vi "ULx Write (Analog 1D DBL 1Chan 1Samp).vi"(0 "task in":refnum<k24>, 1 "auto start":bool=TRUE, 7 "data":dbl, 9 "timeout":dbl=10.0 format="%_4g", 11 "error in":errorcluster) -> (4 "task out":refnum<k24>, 10 "number of samples written per channel":u32, 15 "error out":errorcluster)   [LabVIEW 2020]
doc: "Writes a floating-point sample to a task that contains a single analog output channel."
uses:
  C:/Users/William/Documents/LV 2020 builds/LeaktestDAQ/Source-v33/ULx_LV.dll
  ULx_LV.dll
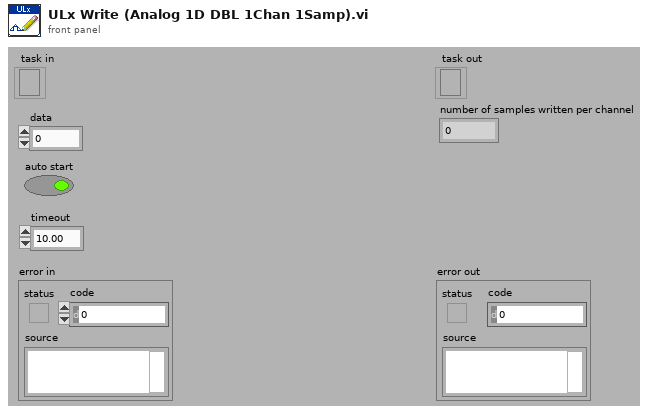
[diagram p1: front panel]
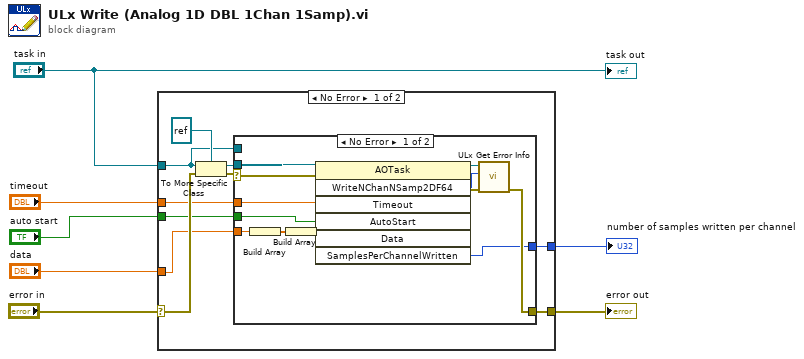
[diagram p0: block diagram]
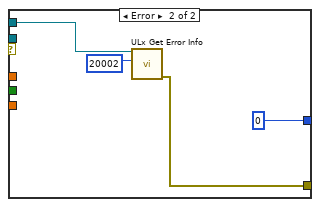
[diagram p2: hidden frame]
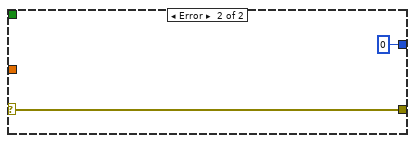
[diagram p3: hidden frame]
diagram:
  n1 = case shown="No Error" "error in" {
    selector: "error in" -> [w17 w35]
    tunnel: "task in" -> [w11 _]
    tunnel: "timeout" -> [w13 _]
    tunnel: [w12 w35] -> w5
    tunnel: "auto start" -> [w10 _]
    tunnel: [w9 0 ("SamplesPerChannelWritten")] -> w2
    tunnel: "data" -> [w8 _]
    frame No Error {
      n2 = To More Specific Class(target class=refnum<k24> refnum, reference=w11, error in=w17) -> (specific class reference=w14:refnum<k24>, error out=w15:errorcluster)
      n3 = case shown="No Error" w15 {
        selector: w15 -> [w28 _]
        tunnel: w14 -> [w29 _]
        tunnel: w13 -> [w22 _]
        tunnel: [w25 w32] -> w12
        tunnel: w11 -> [_ w31]
        tunnel: w10 -> [w21 _]
        tunnel: [w23 0 ("SamplesPerChannelWritten")] -> w9
        tunnel: w8 -> [w20 _]
        frame No Error {
          n4 = Build Array(w20) -> (w18:dbl[])
          n5 = Build Array(w18) -> (w19:dbl[][])
          n6 = invoke class="AOTask" method="WriteNChanNSamp2DF64"(reference=w29, error in=w28, "Timeout"=w22, "AutoStart"=w21, "Data"=w19) -> (reference out=w26:refnum<k24>, error out=w27:errorcluster, "WriteNChanNSamp2DF64"=w24:i32, "SamplesPerChannelWritten"=w23:u32)  [unwired: 2 in, 3 out]
          n7 = call "ULx Get Error Info.vi"("error in"=w27, "ErrorCode"=w24, "task in"=w26) -> ("error out"=w25:errorcluster)  [unwired: 8 in]
        }
        frame Error {
          n8 = call "ULx Get Error Info.vi"("ErrorCode"=20002, "task in"=w31) -> ("error out"=w32:errorcluster)  [unwired: 9 in]
        }
      }
    }
    frame Error {
    }
  }
  "error out" <- w5
  "number of samples written per channel" <- w2
  "task out" <- "task in"
